vi "Create Class.vi"(8 "error in (no error)":errorcluster, 10 "Y-Axis":refnum<class "iMotion Controller.lvclass">, 11 "X-Axis":refnum<class "iMotion Controller.lvclass">) -> (0 "error out":errorcluster, 3 "Sync 2-Axis Stage Controller out":refnum<class "Sync 2-Axis Stage Controller.lvclass">)   [LabVIEW 2022 SP3, in "Sync 2-Axis Stage Controller.lvclass"]
uses:
  Sync 2-Axis Stage Controller.lvclass
  Axis Objects/iMotion Controller/iMotion Controller.lvclass
  Sync 2-Axis Stage Controller.lvclass/Sync 2-Axis Stage Controller.ctl
  Home State.ctl
  <vilib>/ErrorRing/Error Ring.xnode
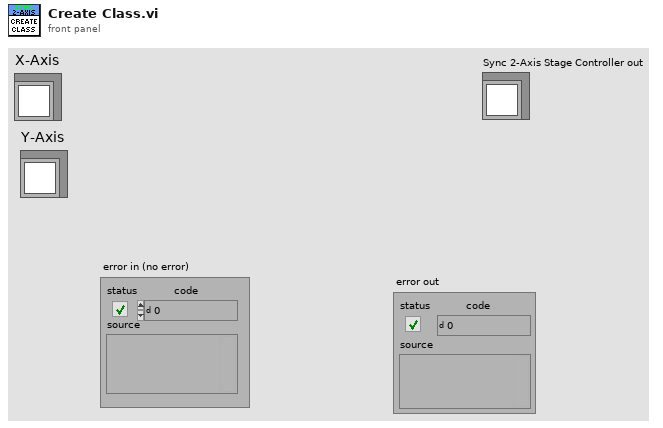
[diagram p1: front panel]
types:
  T1 = typedef "Sync 2-Axis Stage Controller.lvclass/Home State.ctl" = enum16{"Idle", "Homing 1st Axis", "Homing 2nd Axis", "Done"}
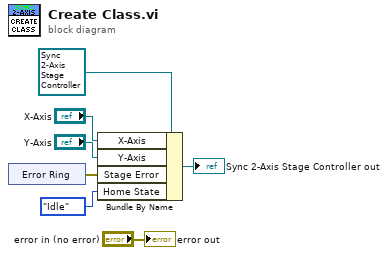
[diagram p0: block diagram]
diagram:
  n1 = xnode "Error Ring"() -> ("error out"=w2:errorcluster)
  n2 = Bundle By Name(cluster=refnum<class "Sync 2-Axis Stage Controller.lvclass"> refnum ("Sync 2-Axis Stage Controller in"), "X-Axis"="X-Axis", "Y-Axis"="Y-Axis", "Stage Error"=w2, "Home State"=Home_State."Idle" ("Enum")) -> (→"Sync 2-Axis Stage Controller out":refnum<class "Sync 2-Axis Stage Controller.lvclass">)
  "error out" <- "error in (no error)"
